vi "create_shared_link.vi"(8 "error in (no error)":errorcluster, 10 "short_url":bool, 11 "path":string) -> (0 "error out":errorcluster, 3 "url":string)   [LabVIEW 2015, in "lv-dropbox.lvlib" / "v2.lvlib"]
uses:
  v2.lvlib
  <vilib>/httpClient/POSTBuffer.vi
  <vilib>/httpClient/LabVIEWHTTPClient.lvlib
  lv-dropbox.lvlib
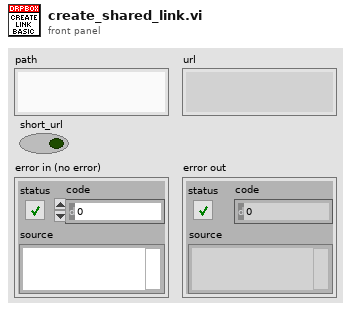
[diagram p1: front panel]
types:
  T1 = cluster{"url":string, "visibility":cluster{".tag":string}, "path":string}
  T2 = typedef "LabVIEWHTTPClient.lvlib/ClientHandle.ctl" = refnum<k1>
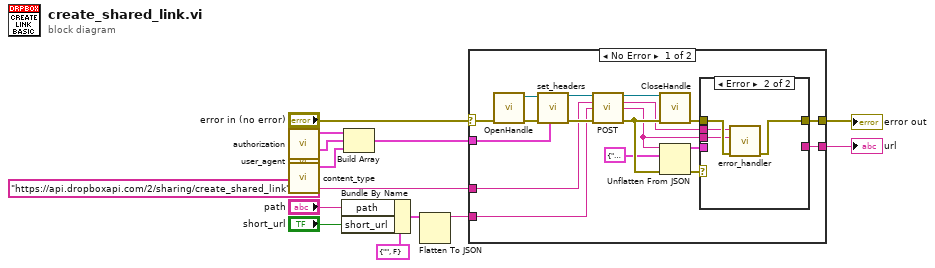
[diagram p0: block diagram]
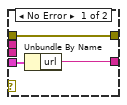
[diagram p2: hidden frame]
diagram:
  n1 = call "authorization.vi"() -> ("header"=w10:cluster{"header":string, "value":string})  [unwired: 11 in]
  n2 = call "user_agent.vi"() -> ("header"=w9:cluster{"header":string, "value":string})  [unwired: 11 in]
  n3 = call "content_type.vi"() -> ("header"=w11:cluster{"header":string, "value":string})  [unwired: 11 in]
  n4 = Bundle By Name(cluster=cluster{"path":string, "short_url":bool} {"path"="", "short_url"=FALSE}, "path"="path", "short_url"="short_url") -> (w4:cluster{"path":string, "short_url":bool})
  n5 = Build Array(w10, w9, w11) -> (w12:cluster{"header":string, "value":string}[])
  n6 = Flatten To JSON(anything=w4) -> (JSON string=w1:string)  [unwired: 2 in, 1 out]
  n7 = case shown="No Error" "error in (no error)" {
    selector: "error in (no error)" -> [w27 w39]
    tunnel: "https://api.dropboxapi.com/2/sharing/create_shared_link" ("url") -> [w29 _]
    tunnel: w12 -> [w25 _]
    tunnel: [w15 w39] -> w8
    tunnel: [w16 _] -> w6
    tunnel: w1 -> [w14 _]
    frame No Error {
      n8 = call <vilib>:"OpenHandle.vi"("error in (no error)"=w27) -> ("client handle out"=w28:T2, "error out"=w26:errorcluster)  [unwired: 13 in]
      n9 = call "set_headers.vi"("header_value []"=w25, "error in (no error)"=w26, "client_handle in"=w28) -> ("error out"=w31:errorcluster, "client_handle out"=w24:T2)  [unwired: 7 in]
      n10 = call-poly <vilib>:"POST.vi"("client handle"=w24, "url"=w29, "buffer"=w14, "error in (no error)"=w31) -> ("client handle out"=w23:T2, "headers"=w17:string, "body"=w18:string, "error out"=w30:errorcluster)  [unwired: 8 in]
      n11 = call <vilib>:"CloseHandle.vi"("client handle"=w23, "error in (no error)"=w30) -> ("error out"=w20:errorcluster)  [unwired: 13 in]
      n12 = Unflatten From JSON(JSON string=w18, type and defaults=T1 {"url"="", "visibility"={".tag"=""}, "path"=""}, error in (no error)=w30) -> (value=w19:T1, error out=w21:errorcluster)  [unwired: 4 in]
      n13 = case shown="Error" w21 {
        tunnel: w20 -> [w34 w38]
        tunnel: [w34 w37] -> w15
        tunnel: w17 -> [_ w36]
        tunnel: w18 -> [_ w35]
        tunnel: w19 -> [w33 _]
        tunnel: [w32 _] -> w16
        frame No Error {
          n14 = Unbundle By Name(w33) -> ("url"=w32:string)
        }
        frame Error {
          n15 = call "error_handler.vi"("error in (no error)"=w38, "body"=w35, "headers"=w36) -> ("error out"=w37:errorcluster)  [unwired: 8 in]
        }
      }
    }
    frame Error {
    }
  }
  "error out" <- w8
  "url" <- w6
